vi "Get9219Properties.vi"(10 "ChannelType":string, 11 "Properties":T2[](array[typedef])) -> (3 "9219 Channel Settings":T1)   [LabVIEW 2017, in "ScanEngine.lvlib"]
uses:
  <vilib>/addons/InsightCM/Devices/Shared/Common/ScanEngine/ScanEngine.lvlib
  <vilib>/addons/InsightCM/MessageBus/Base/controls/KeyValuePair.ctl
  <vilib>/addons/InsightCM/Utilities/PropertyHelpers/PropertyHelpers.lvlib
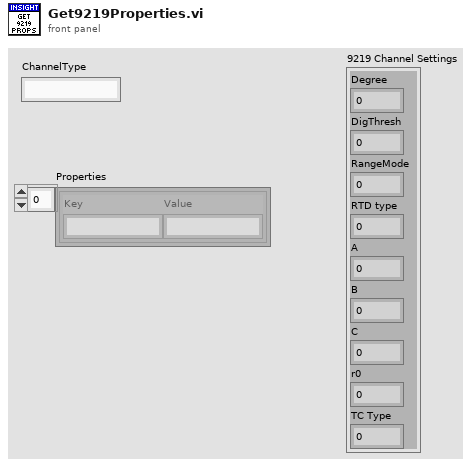
[diagram p1: front panel]
types:
  T1 = cluster{"Degree":u32, "DigThresh":dbl, "RangeMode":u32, "RTD type":u32, "A":dbl, "B":dbl, "C":dbl, "r0":dbl, "TC Type":u32}
  T2 = typedef "KeyValuePair.ctl" = cluster{"Key":string, "Value":string}
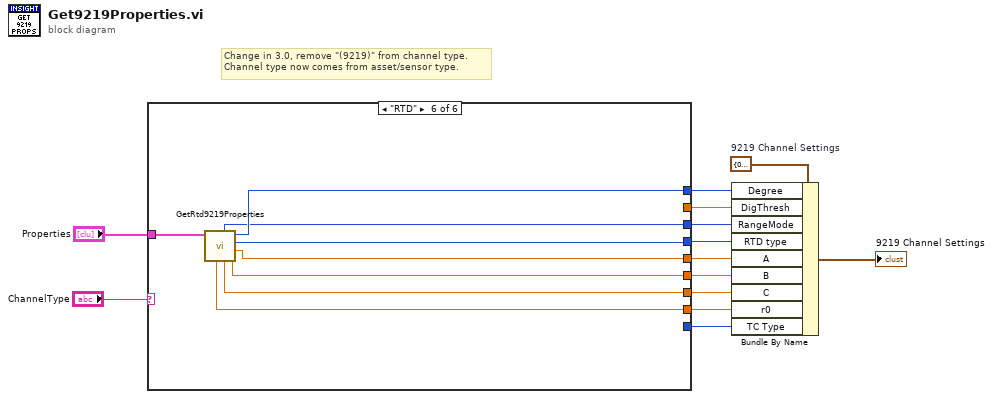
[diagram p0: block diagram]
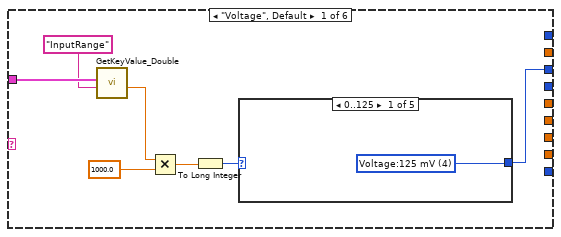
[diagram p2: hidden frame]
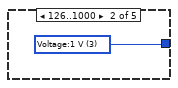
[diagram p3: hidden frame]
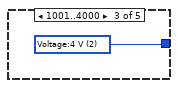
[diagram p4: hidden frame]
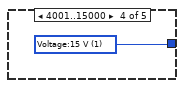
[diagram p5: hidden frame]
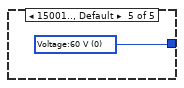
[diagram p6: hidden frame]
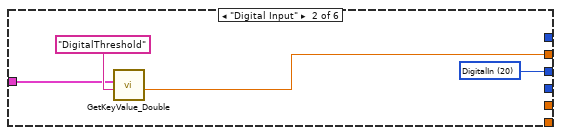
[diagram p7: hidden frame]
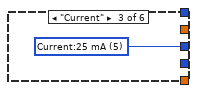
[diagram p8: hidden frame]
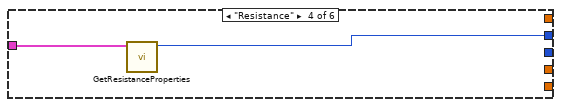
[diagram p9: hidden frame]
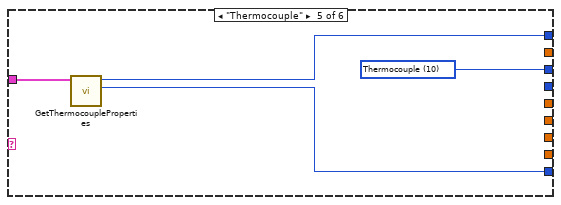
[diagram p10: hidden frame]
diagram:
  w13 = T1 {"Degree"=0, "DigThresh"=0.0, "RangeMode"=11, "RTD type"=0, "A"=0.0, "B"=0.0, "C"=0.0, "r0"=0.0, "TC Type"=0}  # 9219 Channel Settings
  # "Change in 3.0, remove \"(9219)\" from channel type.\nChannel type now comes from asset/sensor type."
  n1 = case shown="\"RTD\"" "ChannelType" {
    tunnel: [_ _ _ _ w34 w44] -> w12
    tunnel: [w17 w29 w30 w31 w36 w37] -> w11
    tunnel: [_ _ _ _ _ w43] -> w10
    tunnel: [_ _ _ _ _ w41] -> w9
    tunnel: [_ _ _ _ _ w40] -> w8
    tunnel: [_ _ _ _ _ w39] -> w7
    tunnel: [_ _ _ _ _ w38] -> w6
    tunnel: [_ _ _ _ w33 _] -> w5
    tunnel: [_ w26 _ _ _ _] -> w3
    tunnel: "Properties" -> [w16 w27 _ w32 w35 w42]
    frame "Voltage", Default {
      n2 = call <vilib>:"GetKeyValue_Double.vi"("key"="InputRange" ("name"), "key value pairs"=w16) -> ("value"=w15:dbl)  [unwired: 7 in, 2 out]
      n3 = Multiply(x=w15, y=1000.0) -> (x*y=w19:dbl)
      n4 = To Long Integer(number=w19) -> (32bit integer=w20:i32)
      n5 = case shown="0..125" w20 {
        tunnel: [w21 w22 w23 w24 w25] -> w17
        frame 0..125 {
          w21 = u32 4 items=["Voltage:60 V", "Voltage:15 V", "Voltage:4 V", "Voltage:1 V", "Voltage:125 mV", "Current:25 mA", "Resistance4W:10 kohms", "Resistance4W:1 kohms", "Resistance2W:10 kohms", "Resistance2W:1 kohms", "Thermocouple", "RTD4W:Pt1000", "RTD4W:Pt100", "RTD3W:Pt1000", "RTD3W:Pt100", "QuarterBridge:350 ohm", "QuarterBridge:120 ohm", "HalfBridge:500 mV/V", "FullBridge:625 mV/V", "FullBridge:78 mV/V", "DigitalIn", "OpenContact"] ("CH0:Range / Mode")
        }
        frame 126..1000 {
          w22 = u32 3 items=["Voltage:60 V", "Voltage:15 V", "Voltage:4 V", "Voltage:1 V", "Voltage:125 mV", "Current:25 mA", "Resistance4W:10 kohms", "Resistance4W:1 kohms", "Resistance2W:10 kohms", "Resistance2W:1 kohms", "Thermocouple", "RTD4W:Pt1000", "RTD4W:Pt100", "RTD3W:Pt1000", "RTD3W:Pt100", "QuarterBridge:350 ohm", "QuarterBridge:120 ohm", "HalfBridge:500 mV/V", "FullBridge:625 mV/V", "FullBridge:78 mV/V", "DigitalIn", "OpenContact"] ("CH0:Range / Mode")
        }
        frame 1001..4000 {
          w23 = u32 2 items=["Voltage:60 V", "Voltage:15 V", "Voltage:4 V", "Voltage:1 V", "Voltage:125 mV", "Current:25 mA", "Resistance4W:10 kohms", "Resistance4W:1 kohms", "Resistance2W:10 kohms", "Resistance2W:1 kohms", "Thermocouple", "RTD4W:Pt1000", "RTD4W:Pt100", "RTD3W:Pt1000", "RTD3W:Pt100", "QuarterBridge:350 ohm", "QuarterBridge:120 ohm", "HalfBridge:500 mV/V", "FullBridge:625 mV/V", "FullBridge:78 mV/V", "DigitalIn", "OpenContact"] ("CH0:Range / Mode")
        }
        frame 4001..15000 {
          w24 = u32 1 items=["Voltage:60 V", "Voltage:15 V", "Voltage:4 V", "Voltage:1 V", "Voltage:125 mV", "Current:25 mA", "Resistance4W:10 kohms", "Resistance4W:1 kohms", "Resistance2W:10 kohms", "Resistance2W:1 kohms", "Thermocouple", "RTD4W:Pt1000", "RTD4W:Pt100", "RTD3W:Pt1000", "RTD3W:Pt100", "QuarterBridge:350 ohm", "QuarterBridge:120 ohm", "HalfBridge:500 mV/V", "FullBridge:625 mV/V", "FullBridge:78 mV/V", "DigitalIn", "OpenContact"] ("CH0:Range / Mode")
        }
        frame 15001.., Default {
          w25 = u32 0 items=["Voltage:60 V", "Voltage:15 V", "Voltage:4 V", "Voltage:1 V", "Voltage:125 mV", "Current:25 mA", "Resistance4W:10 kohms", "Resistance4W:1 kohms", "Resistance2W:10 kohms", "Resistance2W:1 kohms", "Thermocouple", "RTD4W:Pt1000", "RTD4W:Pt100", "RTD3W:Pt1000", "RTD3W:Pt100", "QuarterBridge:350 ohm", "QuarterBridge:120 ohm", "HalfBridge:500 mV/V", "FullBridge:625 mV/V", "FullBridge:78 mV/V", "DigitalIn", "OpenContact"] ("CH0:Range / Mode")
        }
      }
    }
    frame "Digital Input" {
      w29 = u32 20 items=["Voltage:60 V", "Voltage:15 V", "Voltage:4 V", "Voltage:1 V", "Voltage:125 mV", "Current:25 mA", "Resistance4W:10 kohms", "Resistance4W:1 kohms", "Resistance2W:10 kohms", "Resistance2W:1 kohms", "Thermocouple", "RTD4W:Pt1000", "RTD4W:Pt100", "RTD3W:Pt1000", "RTD3W:Pt100", "QuarterBridge:350 ohm", "QuarterBridge:120 ohm", "HalfBridge:500 mV/V", "FullBridge:625 mV/V", "FullBridge:78 mV/V", "DigitalIn", "OpenContact"] ("CH0:Range / Mode")
      n6 = call <vilib>:"GetKeyValue_Double.vi"("key"="DigitalThreshold" ("name"), "key value pairs"=w27) -> ("value"=w26:dbl)  [unwired: 7 in, 2 out]
    }
    frame "Current" {
      w30 = u32 5 items=["Voltage:60 V", "Voltage:15 V", "Voltage:4 V", "Voltage:1 V", "Voltage:125 mV", "Current:25 mA", "Resistance4W:10 kohms", "Resistance4W:1 kohms", "Resistance2W:10 kohms", "Resistance2W:1 kohms", "Thermocouple", "RTD4W:Pt1000", "RTD4W:Pt100", "RTD3W:Pt1000", "RTD3W:Pt100", "QuarterBridge:350 ohm", "QuarterBridge:120 ohm", "HalfBridge:500 mV/V", "FullBridge:625 mV/V", "FullBridge:78 mV/V", "DigitalIn", "OpenContact"] ("9129 Mode")
    }
    frame "Resistance" {
      n7 = call <vilib>:"GetResistanceProperties.vi"("Properties"=w32) -> ("Range Mode"=w31:u32)  [unwired: 10 in]
    }
    frame "Thermocouple" {
      w36 = u32 10 items=["Voltage:60 V", "Voltage:15 V", "Voltage:4 V", "Voltage:1 V", "Voltage:125 mV", "Current:25 mA", "Resistance4W:10 kohms", "Resistance4W:1 kohms", "Resistance2W:10 kohms", "Resistance2W:1 kohms", "Thermocouple", "RTD4W:Pt1000", "RTD4W:Pt100", "RTD3W:Pt1000", "RTD3W:Pt100", "QuarterBridge:350 ohm", "QuarterBridge:120 ohm", "HalfBridge:500 mV/V", "FullBridge:625 mV/V", "FullBridge:78 mV/V", "DigitalIn", "OpenContact"] ("9129 Mode")
      n8 = call <vilib>:"GetThermocoupleProperties.vi"("Properties"=w35) -> ("AI Thermocouple type"=w33:u32, "AI degree range"=w34:u32)  [unwired: 9 in]
    }
    frame "RTD" {
      n9 = call <vilib>:"GetRtd9219Properties.vi"("Properties"=w42) -> ("B"=w40:dbl, "A"=w41:dbl, "RTD type"=w43:u32, "RTD ohm degree range"=w44:u32, "C"=w39:dbl, "Range/Mode"=w37:u32, "r0"=w38:dbl)  [unwired: 4 in]
    }
  }
  n10 = Bundle By Name(cluster=w13, "Degree"=w12, "DigThresh"=w3, "RangeMode"=w11, "RTD type"=w10, "A"=w9, "B"=w8, "C"=w7, "r0"=w6, "TC Type"=w5) -> (→"9219 Channel Settings":T1)
